vi "Write and Provide PES Path.vi"() -> (0 "Error Out":errorcluster, 3 "PES File Path":path)   [LabVIEW 2019, in "OPI.lvclass"]
uses:
  OPI.lvclass
  <vilib>/Utility/sysdir.llb/System Directory Type.ctl
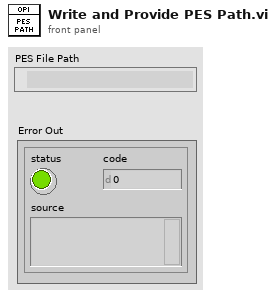
[diagram p1: front panel]
types:
  T1 = enum16{"open", "replace", "create", "open or create", "replace or create", "replace or create with confirmation"}
  T2 = typedef "System Directory Type.ctl" = i32
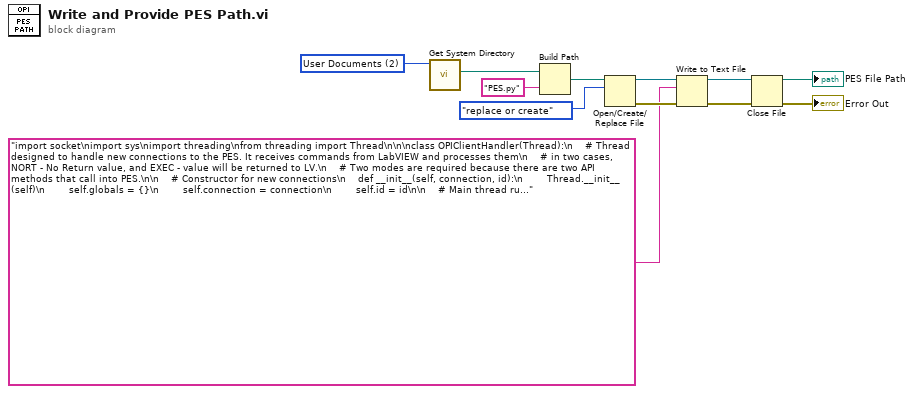
[diagram p0: block diagram]
diagram:
  w12 = T2 2 items=["User Home"=0, "User Desktop"=1, "User Documents"=2, "User Application Data"=3, "User Preferences"=4, "User Temporary"=5, "Public Documents"=6, "Public Application Data"=7, "Public Preferences"=8, "Public Cache"=13, "System Core Libraries"=9, "System Installed Libraries"=10, "Application Files"=11, "Boot Volume Root"=12] ("system directory type")
  n1 = call <vilib>:"Get System Directory.vi"("system directory type"=w12) -> ("system directory"=w10:path)  [unwired: 10 in]
  n2 = Build Path(base path=w10, name or relative path="PES.py") -> (appended path=w9:path)
  n3 = Open/Create/Replace File(file path (use dialog)=w9, operation (0:open)=T1."replace or create") -> (refnum out=w7:refnum<file>, error out=w6:errorcluster)  [unwired: 4 in, 1 out]
  n4 = Write to Text File(file (use dialog)=w7, text="import socket\nimport sys\nimport threading\nfrom threading import Thread\n\n\nclass OPIClientHandler(Thread):\n    # Thread designed to handle new connections to the PES. It receives commands from LabVIEW and processes them\n    # in two cases, NORT - No Return value, and EXEC - value will be returned to LV.\n    # Two modes are required because there are two API methods that call into PES.\n\n    # Constructor for new connections\n    def __init__(self, connection, id):\n        Thread.__init__(self)\n        self.globals = {}\n        self.connection = connection\n        self.id = id\n\n    # Main thread run function with cases to handle commands from LV\n    def run(self):\n        while True:\n            # The size of the command packet is 4 bytes. it defines the behavior of the server.\n            cmnd = self.connection.recv(4)\n\n            if 'EXEC' in str(cmnd):\n                print(\"Handler {0}: Execute command.\".format(self.id))\n                return_exception = \"None\"\n                return_data = \"None\"\n\n                # Receive data from LabVIEW.\n                call = self.receive_data()\n\n                try:\n                    # Try to execute the code provided from LV and send back the return value.\n                    # This locals business is some magic to return the data. Without this it was not working.\n                    loc = locals()\n                    exec(\"return_data\" + str(self.id) + \" = \" + call, self.globals, loc)\n                    return_data = loc['return_data' + str(self.id)]\n                except Exception as e:\n                    # Catch any exceptions raised and send back info to LV.\n                    return_exception = e\n                finally:\n                    # Always send exception data, even if its empty. The protocol requires this.\n                    self.send_data(return_data)\n                    self.send_data(return_exception)\n                    # Return acknowledgement so LV knows there was no error in transmission.\n                    self.connection.sendall(b'OK')\n\n            elif 'NORT' in str(cmnd):\n                print(\"Handler {0}: No Return command.\".format(self.id))\n                return_exception = \"None\"\n\n                # Receive data from LabVIEW.\n                call = self.receive_data()\n\n                try:\n                    # Try to execute the code provided from LV.\n                    exec(call, self.globals)\n                except Exception as e:\n                    # Capture only the exception info\n                    return_exception = e\n                finally:\n                    # Send back exception info. The protocol requires OK back.\n                    self.send_data(return_exception)\n                    # Return acknowledgement so LV knows there was no error in transmission.\n                    self.connection.sendall(b'OK')\n\n            else:\n                # Invalid command sent. The server will shout down\n                print(\"Handler {0}: Invalid cmd or conn closed on client side. Client handler will shut down.\".format(self.id))\n                break\n\n    def send_data(self, data):\n        # Encode data string into bytes\n        bytes_data = str(data).encode(\"ascii\")\n        # Get length of data in bytes\n        data_len = len(bytes_data)\n        # Convert data length to 4 bytes\n        bytes_len = data_len.to_bytes(4, \"big\")\n        # Send the size of string\n        self.connection.sendall(bytes_len)\n        # Send the string itself\n        self.connection.sendall(bytes_data)\n\n    def receive_data(self):\n        # All data transmitted from LabVIEW will be formatted as a string with 4 byte length int in front\n        b = self.connection.recv(4)\n        length = int.from_bytes(b, \"big\", signed=True)\n        # Receive the rest of the message\n        b = self.connection.recv(length)\n        data_string = b.decode(\"ascii\")\n        return data_string\n\n\ndef main():\n    if len(sys.argv) == 2:\n        port = int(sys.argv[1])\n    else:\n        port = 15000\n\n    print(\"Python Execution Server started on localhost port {0}.\".format(port))\n\n    server = socket.socket()\n    server.bind(('localhost', port))\n    server.settimeout(0.01)  # Timeout for listening\n\n    first_conn = False  # Used to check if there was at least one connection made before checking thread numbers\n    stop = False\n    id = 0\n\n    while not stop:\n        try:\n            server.listen(1)\n            (conn, (ip, port)) = server.accept()\n        except socket.timeout:\n            # In case there was a timeout on listening do nothing.\n            pass\n        except:\n            raise\n        else:\n            # If there was no timeout or other exception\n            print(\"New connection established: Handler {0}\".format(id))\n            # Define new thread for OPI client and start\n            new_OPI_client_handler = OPIClientHandler(conn, id)\n            new_OPI_client_handler.start()\n            # Remember that first connection was made and increment ID\n            first_conn = True\n            id += 1\n        finally:\n            # If at least one connection was made and the number of threads == 1, all connections were\n            # stopped and the main server loop can also stop.\n            if first_conn:\n                if len(threading.enumerate()) == 1:\n                    print(\"All connections closed. Server will shut down.\")\n                    stop = True\n\n    server.close()\n\nmain()" ("name or relative path"), error in=w6) -> (refnum out=w4:refnum<file>, error out=w3:errorcluster)  [unwired: 1 in, 1 out]
  n5 = Close File(refnum=w4, error in=w3) -> (path=→"PES File Path":path, error out=→"Error Out":errorcluster)
